vi "多帧发送机制(EV05).vi"(0 "can卡类型":u8, 1 "设备索引号":u8, 2 "CAN端口":u8, 3 "命令":u8 format="%x", 4 "板号":u8 format="%x", 5 "命令序号":u32, 6 "输入数据":dbl[](array[numeric]), 7 "错误输入（无错误）":errorcluster, 10 "流控帧":refnum<vi>) -> (14 "错误代码":u32, 15 "总发送帧数":i32, 19 "错误输出":errorcluster)   [LabVIEW 2013]
panel:
  out "发送成功":bool
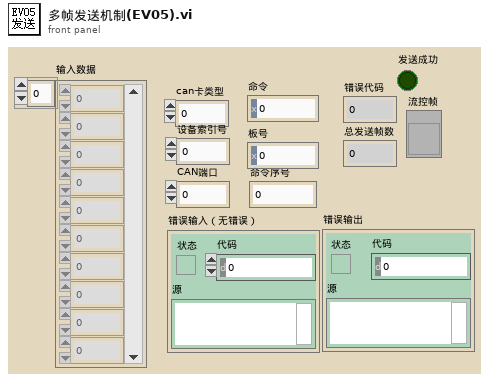
[diagram p1: front panel]
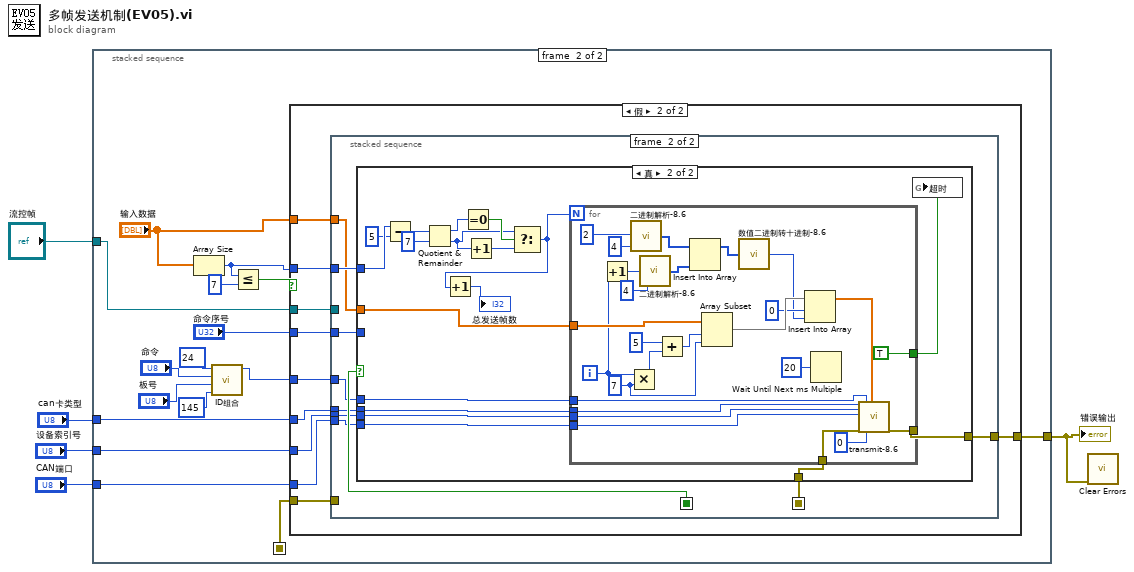
[diagram p0: block diagram]
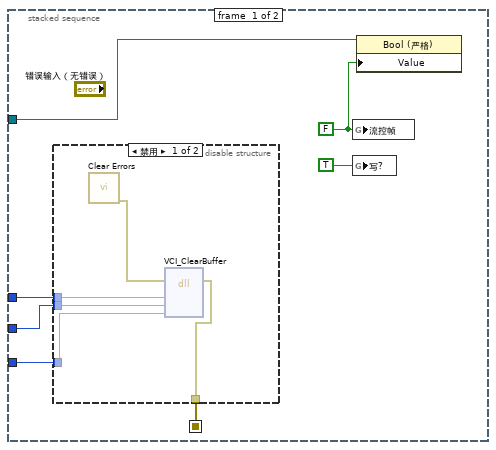
[diagram p2: hidden frame]
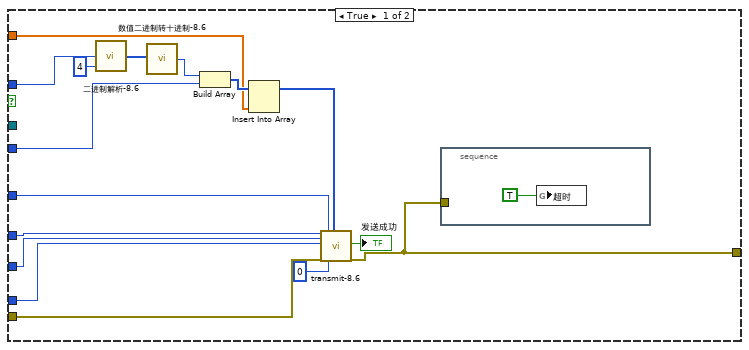
[diagram p4: hidden frame]
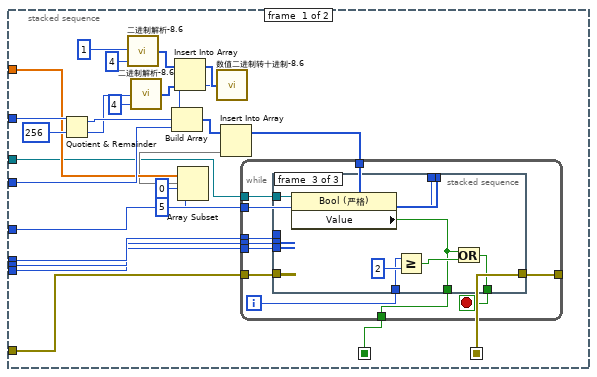
[diagram p5: hidden frame]
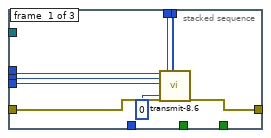
[diagram p6: hidden frame]
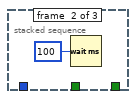
[diagram p7: hidden frame]
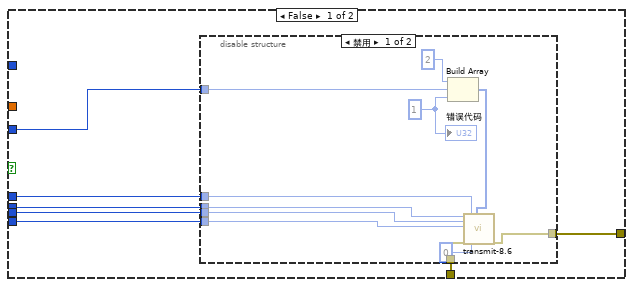
[diagram p8: hidden frame]
diagram:
  n1 = stacked-sequence {
    seq-local: [w9 _] -> [_ w25]
    tunnel: "can卡类型" -> [w12 w28]
    tunnel: "设备索引号" -> [w11 w27]
    tunnel: "CAN端口" -> [w10 w26]
    tunnel: [_ w24] -> w2
    tunnel: "流控帧" -> [w7 w18]
    frame #0 {
      w6 = FALSE ("流控帧")
      n2 = disable-structure shown="禁用" {
        disable-tunnel: w12 -> [w17 _]
        disable-tunnel: w11 -> [w16 _]
        disable-tunnel: w10 -> [w15 _]
        disable-tunnel: [w14 _] -> w9
        frame Disabled {
          n3 = call <vilib>:"Clear Errors.vi"() -> ("error out"=w13:errorcluster)  [unwired: 1 in, 6 out]
          n4 = dll-call lib="PTH1abs FBluewave New EnergySVN_WorkAutoTest_TestStandtrunkAutoTest_TestStandDriverZlgCanBHN01è¯»ååæ°data\nkerneldlls\nusbcan.dll" fn="VCI_ClearBuffer"(error in=w13, "DeviceType"=w17, "DeviceInd"=w16, "CANInd"=w15) -> (error out=w14:errorcluster)  [unwired: 2 in, 5 out]
        }
        frame Enabled {
        }
      }
      n5 = global write "EV05全局变量1.vi" "流控帧"(w6) -> ()
      n6 = global write "EV05全局变量1.vi" "写?"(TRUE ("写?")) -> ()
      n7 = property class="Bool (严格)"(reference=w7, "Value"=w6) -> ()  [unwired: 1 in, 2 out]
    }
    frame #1 {
      n8 = Array Size(array="输入数据") -> (size(s)=w31:i32)
      n9 = call "ID组合.vi"("SA(4)"=145 ("PDU(1)"), "PS(3)"="板号", "PF(2)"="命令", "PDU(1)"=24) -> ("ID"=w19:i32)  [unwired: 7 out]
      n10 = Less Or Equal?(x=w31, y=7) -> (x <= y?=w32:bool)
      n11 = case shown="假" w32 {
        tunnel: w28 -> [w49 w60]
        tunnel: w27 -> [w48 w59]
        tunnel: w26 -> [w47 w58]
        tunnel: w31 -> [w45 w55]
        tunnel: "命令序号" -> [w46 w57]
        tunnel: "输入数据" -> [w40 w54]
        tunnel: w19 -> [w36 w56]
        tunnel: w25 -> [w38 w53]
        tunnel: [w37 w52] -> w24
        tunnel: w18 -> [_ w51]
        frame True {
          n12 = call "二进制解析-8.6.vi"("索引"=4, "数值"=w45) -> ("低位子数组"=w43:i32[])  [unwired: 3 out]
          n13 = call "数值二进制转十进制-8.6.vi"("子数组"=w43) -> ("十进制数值"=w42:i32)  [unwired: 4 out]
          n14 = Build Array(w42, w46) -> (w41:u32[])
          n15 = Insert Into Array(array=w41, new element=w40) -> (w39:u32[])  [unwired: 1 in]
          n16 = call "transmit-8.6.vi"("can卡类型"=w49, "设备索引号"=w48, "CAN端口"=w47, "错误输入（无错误）"=w38, "ID"=w36, "SendType"=u8 0, "Data"=w39) -> ("发送成功"=→"发送成功":bool, "错误输出"=w37:errorcluster)  [unwired: 2 in, 9 out]
          n17 = stacked-sequence {
            tunnel: w37 -> [_]
            frame #0 {
              n18 = global write "EV05全局变量1.vi" "超时"(TRUE ("超时")) -> ()
            }
          }
        }
        frame False {
          n19 = stacked-sequence {
            seq-local: [w62 _] -> [_ w122]
            seq-local: [w64 _] -> [_ w115]
            tunnel: w60 -> [w86 w118]
            tunnel: w59 -> [w85 w117]
            tunnel: w58 -> [w84 w116]
            tunnel: w57 -> [w83 w113]
            tunnel: w56 -> [w80 w119]
            tunnel: w55 -> [w79 w121]
            tunnel: w54 -> [w69 w120]
            tunnel: w53 -> [w65 _]
            tunnel: [_ w114] -> w52
            tunnel: w51 -> [w61 _]
            frame #0 {
              n20 = Quotient & Remainder(x=w79, y=256) -> (x-y*floor(x/y)=w77:i32, floor(x/y)=w76:i32)
              n21 = call "二进制解析-8.6.vi"("索引"=4, "数值"=1) -> ("低位子数组"=w63:i32[])  [unwired: 3 out]
              n22 = call "二进制解析-8.6.vi"("索引"=4, "数值"=w76) -> ("低位子数组"=w72:i32[])  [unwired: 3 out]
              n23 = Insert Into Array(array=w63, new element=w72) -> (w71:i32[])  [unwired: 1 in]
              n24 = Array Subset(array=w69, index=0 ("索引"), length=5 ("长度")) -> (w66:dbl[])
              n25 = call "数值二进制转十进制-8.6.vi"("子数组"=w71) -> ("十进制数值"=w70:i32)  [unwired: 4 out]
              n26 = Build Array(w70, w77, w83) -> (w82:u32[])
              n27 = Insert Into Array(array=w82, new element=w66) -> (w81:u32[])  [unwired: 1 in]
              n28 = while {
                tunnel: w86 -> [w97]
                tunnel: w85 -> [w96]
                tunnel: w84 -> [w95]
                tunnel: w81 -> [w94]
                tunnel: w80 -> [w93]
                tunnel: [w88] -> w62
                tunnel: w65 -> [w92]
                tunnel: [w91] -> w64
                tunnel: w61 -> [w87]
                i -> [w90]
                stop <- w89 stop-if-true
                n29 = stacked-sequence {
                  tunnel: w97 -> [w105 _ _]
                  tunnel: w96 -> [w104 _ _]
                  tunnel: w95 -> [w103 _ _]
                  tunnel: w94 -> [w102 _ _]
                  tunnel: w93 -> [w101 _ _]
                  tunnel: w92 -> [w100 _ _]
                  tunnel: [w99 _ _] -> w91
                  tunnel: w90 -> [_ _ w111]
                  tunnel: [_ _ w109] -> w89
                  tunnel: [_ _ w107] -> w88
                  tunnel: w87 -> [_ _ w108]
                  frame #0 {
                    n30 = call "transmit-8.6.vi"("can卡类型"=w105, "设备索引号"=w104, "CAN端口"=w103, "错误输入（无错误）"=w100, "ID"=w101, "SendType"=u8 0, "Data"=w102) -> ("错误输出"=w99:errorcluster)  [unwired: 2 in, 10 out]
                  }
                  frame #1 {
                    n31 = Wait (ms)(milliseconds to wait=u32 100 ("等待时间（毫秒）")) -> ()  [unwired: 1 out]
                  }
                  frame #2 {
                    n32 = property class="Bool (严格)"(reference=w108) -> ("Value"=w107:bool)  [unwired: 1 in, 2 out]
                    n33 = Greater Or Equal?(x=w111, y=2) -> (x >= y?=w110:bool)
                    n34 = Or(x=w107, y=w110) -> (x .or. y?=w109:bool)
                  }
                }
              }
            }
            frame #1 {
              n35 = case shown="真" w122 {
                tunnel: w121 -> [_ w158]
                tunnel: w120 -> [_ w150]
                tunnel: w119 -> [w123 w149]
                tunnel: w118 -> [w127 w148]
                tunnel: w117 -> [w126 w147]
                tunnel: w116 -> [w125 w146]
                tunnel: w115 -> [w129 w145]
                tunnel: [w128 w144] -> w114
                tunnel: w113 -> [w124 _]
                frame False {
                  n36 = disable-structure shown="禁用" {
                    disable-tunnel: w129 -> [w140 _]
                    disable-tunnel: [w139 _] -> w128
                    disable-tunnel: w127 -> [w138 _]
                    disable-tunnel: w126 -> [w137 _]
                    disable-tunnel: w125 -> [w136 _]
                    disable-tunnel: w124 -> [w133 _]
                    disable-tunnel: w123 -> [w131 _]
                    frame Disabled {
                      w132 = u32 1 ("元素")
                      n37 = Build Array(u8 2 ("元素"), w133, w132) -> (w134:u32[])
                      n38 = call "transmit-8.6.vi"("can卡类型"=w138, "设备索引号"=w137, "CAN端口"=w136, "错误输入（无错误）"=w140, "ID"=w131, "SendType"=u8 0, "Data"=w134) -> ("错误输出"=w139:errorcluster)  [unwired: 2 in, 10 out]
                      "错误代码" <- w132
                    }
                    frame Enabled {
                    }
                  }
                }
                frame True {
                  n39 = Subtract(x=w158, y=5) -> (x-y=w156:i32)
                  n40 = Quotient & Remainder(x=w156, y=7) -> (x-y*floor(x/y)=w154:i32, floor(x/y)=w152:i32)
                  n41 = Equal To 0?(x=w154) -> (x = 0?=w153:bool)
                  n42 = Increment(x=w152) -> (x+1=w151:i32)
                  n43 = Select(t=w152, s=w153, f=w151) -> (s? t:f=w143:i32)
                  n44 = Increment(x=w143) -> (x+1=→"总发送帧数":i32)
                  n45 = for {
                    N: w143 -> [_]
                    tunnel: w150 -> [w181]
                    tunnel: w149 -> [w170]
                    tunnel: w148 -> [w169]
                    tunnel: w147 -> [w168]
                    tunnel: w146 -> [w167]
                    tunnel: w145 -> [w166]
                    tunnel: [w165] -> w144
                    tunnel: [TRUE] -> w141
                    i -> [w179]
                    w176 = 7 ("y")
                    n46 = Increment(x=w179) -> (x+1=w184:i32)
                    n47 = Multiply(x=w179, y=w176) -> (x*y=w178:i32)
                    n48 = call "二进制解析-8.6.vi"("索引"=4, "数值"=2) -> ("低位子数组"=w160:i32[])  [unwired: 3 out]
                    n49 = call "二进制解析-8.6.vi"("索引"=4, "数值"=w184) -> ("低位子数组"=w182:i32[])  [unwired: 3 out]
                    n50 = Add(x=5 ("索引"), y=w178) -> (x+y=w177:i32)
                    n51 = Insert Into Array(array=w160, new element=w182) -> (w175:i32[])  [unwired: 1 in]
                    n52 = Array Subset(array=w181, index=w177, length=w176) -> (w174:dbl[])
                    n53 = call "数值二进制转十进制-8.6.vi"("子数组"=w175) -> ("十进制数值"=w172:i32)  [unwired: 4 out]
                    n54 = Insert Into Array(array=w174, index=0 ("索引"), new element=w172) -> (w171:dbl[])
                    n55 = Wait Until Next ms Multiple(millisecond multiple=u32 20 ("毫秒倍数")) -> ()  [unwired: 1 out]
                    n56 = call "transmit-8.6.vi"("can卡类型"=w169, "设备索引号"=w168, "CAN端口"=w167, "错误输入（无错误）"=w166, "ID"=w170, "SendType"=u8 0, "Data"=w171) -> ("错误输出"=w165:errorcluster)  [unwired: 2 in, 10 out]
                  }
                  n57 = global write "EV05全局变量1.vi" "超时"(w141) -> ()
                }
              }
            }
          }
        }
      }
    }
  }
  "错误输出" <- w2
  n58 = call <vilib>:"Clear Errors.vi"("error in (no error)"=w2) -> ()  [unwired: 7 out]
